vi "Positions2MultiList.vi"(8 "error in (no error)":errorcluster, 11 "Saved Positions":T1(array[cluster])) -> (0 "error out":errorcluster, 3 "Array":string[][](array[string]))   [LabVIEW 2018]
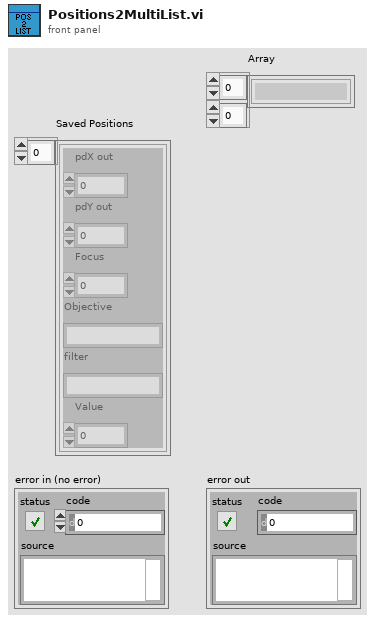
[diagram p1: front panel]
types:
  T1 = cluster{"pdX out":dbl, "pdY out":dbl, "Focus":dbl, "Objective":string, "filter":string, "Value":dbl}[]
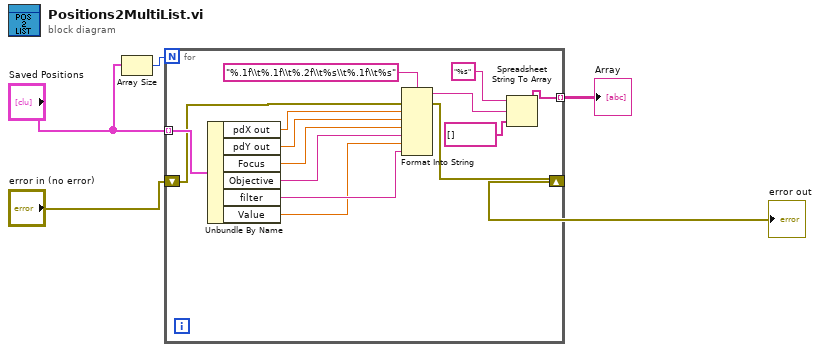
[diagram p0: block diagram]
diagram:
  n1 = Array Size(array="Saved Positions") -> (size(s)=w2:i32)
  n2 = for {
    N: w2 -> [_]
    tunnel: "Saved Positions" -> [w19] mode=indexing
    tunnel: [w9] -> w5 mode=indexing
    shift-right: [w12] -> w4
    shift-left: "error in (no error)" -> [w14]
    n3 = Unbundle By Name(w19) -> ("pdX out"=w18:dbl, "pdY out"=w17:dbl, "Focus"=w16:dbl, "Objective"=w15:string, "filter"=w7:string, "Value"=w6:dbl)
    n4 = Format Into String(format string="%.1f\\t%.1f\\t%.2f\\t%s\\t%.1f\\t%s", error in=w14, w18, w17, w16, w15, w6, w7) -> (resulting string=w11:string, error out=w12:errorcluster)  [unwired: 1 in]
    n5 = Spreadsheet String To Array(format string="%s", spreadsheet string=w11, array type (2D Dbl)=string[] []) -> (array=w9:string[])  [unwired: 1 in]
  }
  "Array" <- w5
  "error out" <- w4
